vi "CalcMeasureTimeInSeconds.vi"(8 "error in (no error)":errorcluster, 9 "exposure_time_in_ms":dbl, 10 "nob":u32, 11 "nos":u32=6) -> (0 "error out":errorcluster, 3 "measureTimeInSeconds":dbl=255.0)   [LabVIEW 2015, in "ESLSCDLL.lvlib"]
uses:
  ESLSCDLL.lvlib
  Globals.vi
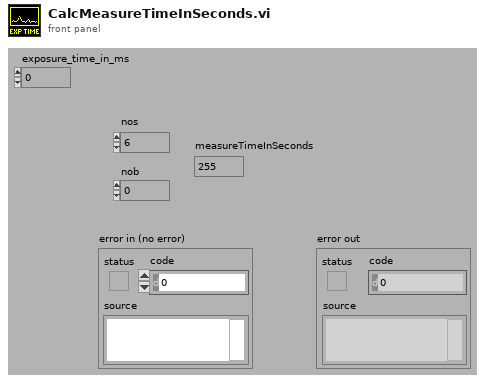
[diagram p1: front panel]
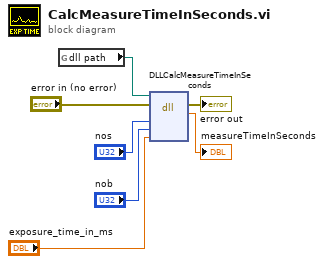
[diagram p0: block diagram]
diagram:
  n1 = global read "Globals.vi" "dll path"() -> (w1:path)
  n2 = dll-call lib="C:/ENTW/PCIE/LV64/board.vis/ESLSCDLL.dll" fn="DLLCalcMeasureTimeInSeconds" ("lwlscdll.dll:DLLReadLongS0")(path in=w1, error in="error in (no error)", "nos"="nos", "nob"="nob", "exposure_time_in_ms"="exposure_time_in_ms") -> (error out=→"error out":errorcluster, "Rückgabetyp"=→"measureTimeInSeconds":dbl)  [unwired: 4 in, 1 out]
